vi "RenameAndRemove.vi"(0 "ClassName":string, 1 "ClassRefnum":refnum<vi>, 2 "TemplateFolder":path, 3 "TemplateName":string, 5 "error in":errorcluster) -> (14 "ViRefsOut":refnum<vi>[](array[refnum]), 15 "DeleteFiles":path[](array[path]), 17 "ItemLocked":bool[](array[boolean]), 18 "Items":refnum<vi>[](array[refnum]), 19 "error out":errorcluster)   [LabVIEW 2020, in "ClassWriterGOOP400.lvclass"]
uses:
  <resource>/Framework/Providers/Open_GDS/ClassProviders/Provider_EndevoGOOP400/ClassWriterGOOP400_class/ClassWriterGOOP400.lvclass
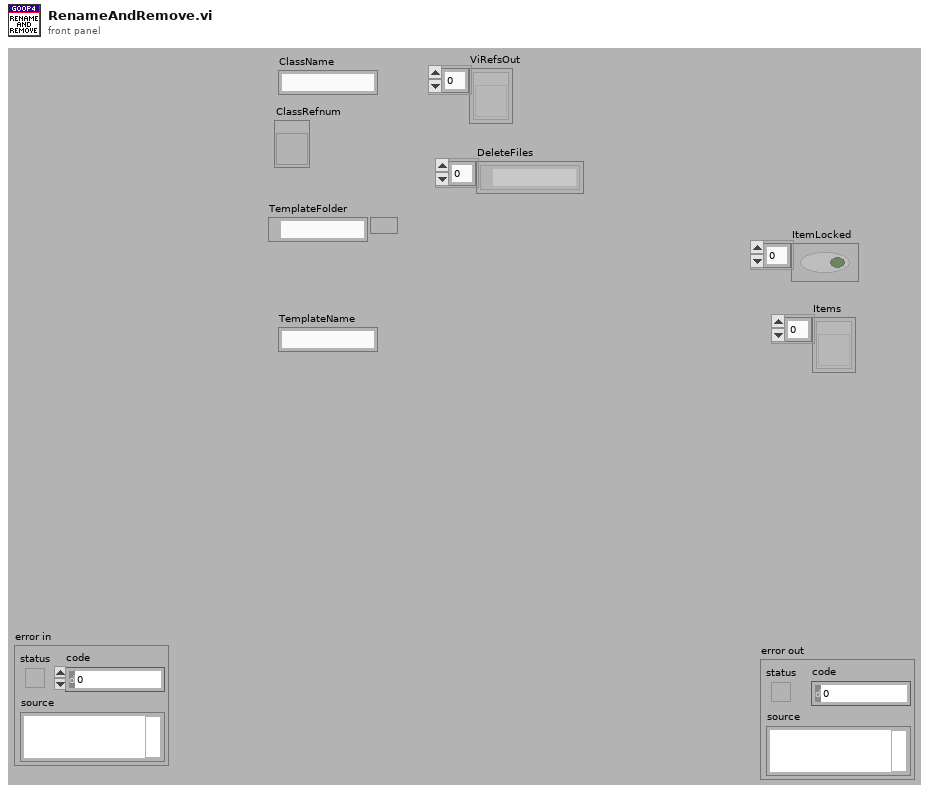
[diagram p1: front panel]
types:
  T1 = enum32{"invalid lock state", "Not Locked", "Locked (No Password)", "Password-protected"}
  T2 = enum32{"invalid scope", "public", "private", "protected", "community"}
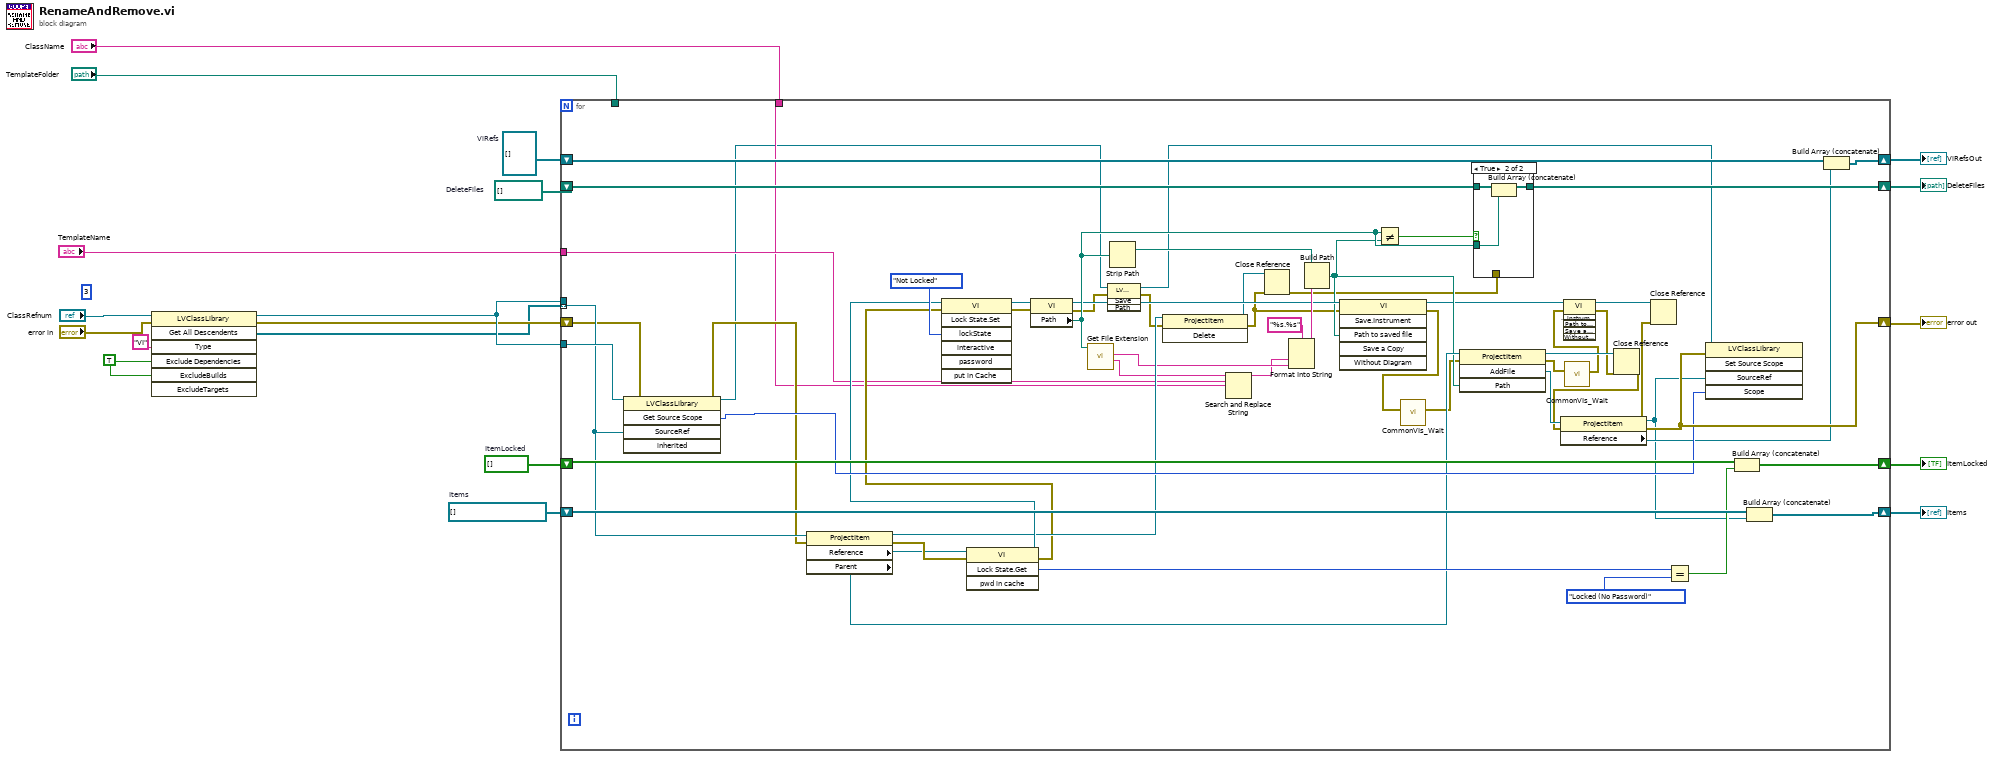
[diagram p0: block diagram]
diagram:
  w1 = TRUE ("ExcludeDependencies")
  (unwired) 3
  w18 = path[] []  # DeleteFiles
  w16 = bool[] []  # ItemLocked
  w14 = refnum<vi>[] []  # Items
  w7 = refnum<vi>[] []  # ViRefs
  n1 = invoke class="LVClassLibrary" method="Get All Descendents"(reference="ClassRefnum", error in="error in", "Type"="VI", "Exclude Dependencies"=w1, "ExcludeBuilds"=w1) -> (reference out=w19:refnum<vi>, error out=w5:errorcluster, "All Descendents"=w3:refnum<vi>[])  [unwired: 2 in, 4 out]
  n2 = for {
    shift-right: [w74] -> w8
    shift-left: w7 -> [w75]
    shift-right: [w76] -> w11
    shift-left: w5 -> [w28]
    tunnel: "ClassName" -> [w29]
    tunnel: "TemplateFolder" -> [_]
    shift-right: [w73] -> w10
    shift-left: w18 -> [w72]
    tunnel: w3 -> [w66] mode=indexing
    tunnel: w19 -> [_]
    shift-right: [w70] -> w15
    shift-left: w14 -> [w71]
    shift-right: [w69] -> w17
    shift-left: w16 -> [w68]
    tunnel: w19 -> [w67]
    tunnel: "TemplateName" -> [w30]
    n3 = invoke class="LVClassLibrary" method="Get Source Scope"(reference=w67, error in=w28, "SourceRef"=w66) -> (reference out=w27:refnum<vi>, error out=w64:errorcluster, "GetSourceScope"=w65:T2)  [unwired: 2 in, 2 out]
    n4 = property class="ProjectItem"(reference=w66, error in=w64) -> (reference out=w50:refnum<vi>, error out=w62:errorcluster, "Reference"=w58:refnum<vi>, "Parent"=w52:refnum<vi>)
    n5 = invoke class="VI" method="Lock State.Get"(reference=w58, error in=w62) -> (reference out=w56:refnum<vi>, error out=w42:errorcluster, "Get Lock State"=w61:T1)  [unwired: 2 in, 1 out]
    n6 = invoke class="VI" method="Lock State.Set"(reference=w56, error in=w42, "lockState"=T1."Not Locked" ("Lock State")) -> (reference out=w45:refnum<vi>, error out=w44:errorcluster)  [unwired: 4 in, 5 out]
    n7 = property class="VI"(reference=w45, error in=w44) -> (reference out=w48:refnum<vi>, error out=w25:errorcluster, "Path"=w54:path)
    n8 = call <vilib>:"Get File Extension.vi"("file"=w54) -> ("filename without extension"=w31:string, "lowercase file extension"=w33:string)  [unwired: 6 in, 3 out]
    n9 = invoke class="LVClassLibrary" method="Save"(reference=w27, error in=w25) -> (reference out=w26:refnum<vi>, error out=w24:errorcluster)  [unwired: 2 in, 2 out]
    n10 = Strip Path(path=w54) -> (stripped path=w53:path)  [unwired: 1 out]
    n11 = invoke class="ProjectItem" method="Delete"(reference=w50, error in=w24) -> (reference out=w40:refnum<vi>, error out=w41:errorcluster)  [unwired: 1 in, 1 out]
    n12 = Search and Replace String(input string=w31, search string=w30, replace string=w29) -> (result string=w32:string)  [unwired: 5 in, 3 out]
    n13 = Close Reference(reference=w40, error in (no error)=w41) -> (error out=w34:errorcluster)
    n14 = Format Into String(format string="%s.%s", w32, w33) -> (resulting string=w51:string)  [unwired: 2 in, 1 out]
    n15 = Build Path(base path=w53, name or relative path=w51) -> (appended path=w47:path)
    n16 = invoke class="VI" method="Save.Instrument"(reference=w48, error in=w41, "Path to saved file"=w47) -> (reference out=w38:refnum<vi>, error out=w21:errorcluster)  [unwired: 3 in, 4 out]
    n17 = Not Equal?(x=w54, y=w47) -> (x != y?=w55:bool)
    n18 = call <resource>:"CommonVIs_Wait.vi"("error in"=w21) -> ("error out"=w20:errorcluster)  [unwired: 9 in]
    n19 = invoke class="ProjectItem" method="AddFile"(reference=w52, error in=w20, "Path"=w47) -> (reference out=w39:refnum<vi>, error out=w23:errorcluster, "AddFile"=w49:refnum<vi>)  [unwired: 1 in, 1 out]
    n20 = case shown="True" w55 {
      tunnel: w54 -> [_ w78]
      tunnel: w72 -> [w77 w80]
      tunnel: [w77 w79] -> w73
      tunnel: w34 -> [_ _]
      frame False {
      }
      frame True {
        n21 = Build Array (concatenate)(w80, w78) -> (w79:path[])
      }
    }
    n22 = call <resource>:"CommonVIs_Wait.vi"("error in"=w23) -> ("error out"=w22:errorcluster)  [unwired: 9 in]
    n23 = invoke class="VI" method="Save.Instrument"(reference=w38, error in=w22) -> (reference out=w35:refnum<vi>, error out=w37:errorcluster)  [unwired: 4 in, 4 out]
    n24 = Close Reference(reference=w39, error in (no error)=w37) -> (error out=w36:errorcluster)
    n25 = property class="ProjectItem"(reference=w49, error in=w36) -> (reference out=w43:refnum<vi>, error out=w76:errorcluster, "Reference"=w46:refnum<vi>)
    n26 = Close Reference(reference=w35, error in (no error)=w76) -> ()  [unwired: 1 out]
    n27 = Equal?(x=w61, y=T1."Locked (No Password)") -> (x = y?=w59:bool)
    n28 = invoke class="LVClassLibrary" method="Set Source Scope"(reference=w26, error in=w76, "SourceRef"=w43, "Scope"=w65) -> ()  [unwired: 1 in, 5 out]
    n29 = Build Array (concatenate)(w68, w59) -> (w69:bool[])
    n30 = Build Array (concatenate)(w71, w43) -> (w70:refnum<vi>[])
    n31 = Build Array (concatenate)(w75, w46) -> (w74:refnum<vi>[])
  }
  "ItemLocked" <- w17
  "Items" <- w15
  "error out" <- w11
  "DeleteFiles" <- w10
  "ViRefsOut" <- w8
